vi "ini.vi"() -> (2 "Array 2":dbl[][](array[numeric]))   [LabVIEW 2020]
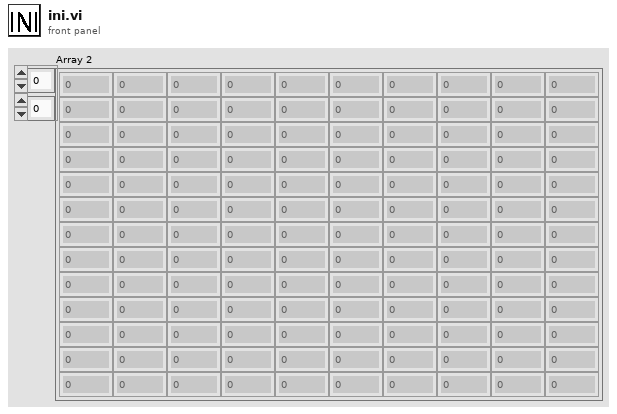
[diagram p1: front panel]
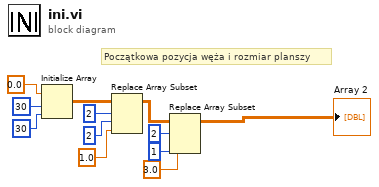
[diagram p0: block diagram]
diagram:
  # "Początkowa pozycja węża i rozmiar planszy"
  n1 = Initialize Array(0.0 ("element"), 30 ("dimension size"), 30 ("dimension size")) -> (w9:dbl[][])
  n2 = Replace Array Subset(array=w9, new element=1.0 ("new element/subarray"), index (row)=2, index (col)=2 ("disabled index (col)")) -> (w5:dbl[][])
  n3 = Replace Array Subset(array=w5, new element=3.0 ("new element/subarray"), index (row)=2, index (col)=1 ("disabled index (col)")) -> (→"Array 2":dbl[][])
